vi "Generate mounth year strings.vi"(7 "Dashes?":bool, 11 "seconds since 1904 (default 0 = now)":u32) -> (0 "mmdd":string, 2 "hhmmss_mmdd":string, 3 "Month_year":string)   [LabVIEW 2015]
panel:
  out "Old result":string
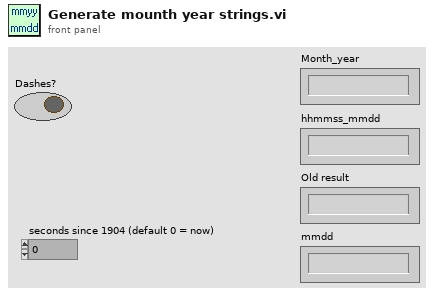
[diagram p1: front panel]
types:
  T1 = typedef "LVDateTimeRec.ctl" = cluster{"fractional second":dbl, "second":i32, "minute":i32, "hour":i32, "day of month":i32, "month":i32, "year":i32, "day of week":i32, "day of year":i32, "DST":i32}
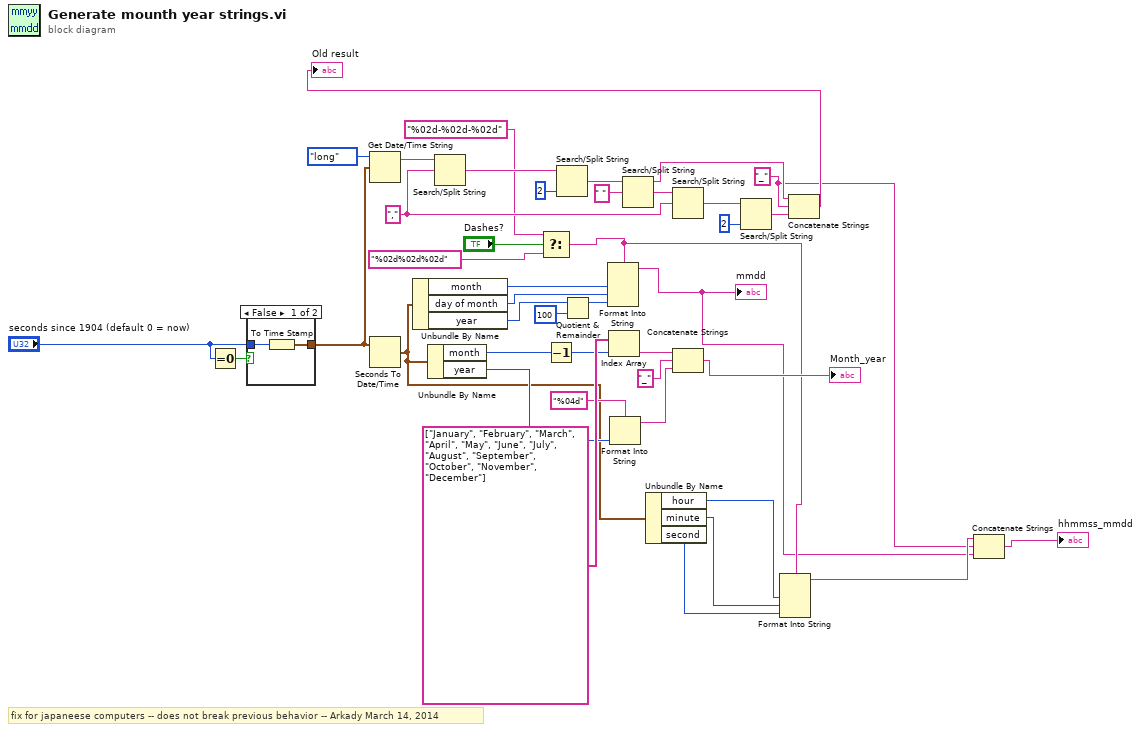
[diagram p0: block diagram]
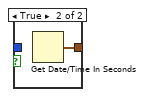
[diagram p2: hidden frame]
diagram:
  w2 = "_" ("substring before char")
  w34 = ","
  # "fix for japaneese computers -- does not break previous behavior -- Arkady March 14, 2014"
  n1 = Equal To 0?(x="seconds since 1904 (default 0 = now)") -> (x = 0?=w31:bool)
  n2 = case shown="False" w31 {
    tunnel: [w43 w45] -> w25
    tunnel: "seconds since 1904 (default 0 = now)" -> [w44 _]
    frame False {
      n3 = To Time Stamp(1:w44) -> (0:w43:timestamp)
    }
    frame True {
      n4 = Get Date/Time In Seconds() -> (seconds since 1Jan1904=w45:timestamp)
    }
  }
  n5 = Get Date/Time String(date format (0)=enum16{"short", "long", "abbreviated"}."long", seconds (now)=w25) -> (date string=w42:string)  [unwired: 2 out]
  n6 = Seconds To Date/Time(time stamp (now)=w25) -> (date time rec=w9:T1)  [unwired: 1 out]
  n7 = Unbundle By Name(w9) -> ("month"=w29:i32, "day of month"=w28:i32, "year"=w13:i32)
  n8 = Unbundle By Name(w9) -> ("month"=w15:i32, "year"=w12:i32)
  n9 = Search/Split String(string=w42, search string/char (-)=w34) -> (match + rest of string=w40:string)  [unwired: 3 out]
  n10 = Select(t="%02d-%02d-%02d", s="Dashes?", f="%02d%02d%02d") -> (s? t:f=w8:string)
  n11 = Decrement(x=w15) -> (x-1=w14:i32)
  n12 = Search/Split String(string=w40, offset (0)=2) -> (match + rest of string=w39:string)  [unwired: 3 out]
  n13 = Quotient & Remainder(x=w13, y=100) -> (x-y*floor(x/y)=w26:i32)  [unwired: 1 out]
  n14 = Format Into String(format string=w8, w29, w28, w26) -> (resulting string=w3:string)  [unwired: 2 in, 1 out]
  "mmdd" <- w3
  n15 = Index Array(array=string[] ["January", "February", "March", "April", "May", "June", "July", "August", "September", "October", "November", "December"], index=w14) -> (element=w18:string)
  n16 = Format Into String(format string="%04d", w12) -> (resulting string=w16:string)  [unwired: 2 in, 1 out]
  n17 = Search/Split String(string=w39, search string/char (-)=" ") -> (substring before match=w32:string, match + rest of string=w36:string)  [unwired: 2 out]
  n18 = Unbundle By Name(w9) -> ("hour"=w7:i32, "minute"=w6:i32, "second"=w5:i32)
  n19 = Search/Split String(string=w36, search string/char (-)=w34) -> (match + rest of string=w33:string)  [unwired: 3 out]
  n20 = Concatenate Strings(w18, "_" ("substring before char"), w16) -> (→"Month_year":string)
  n21 = Search/Split String(string=w33, offset (0)=2) -> (match + rest of string=w37:string)  [unwired: 3 out]
  n22 = Format Into String(format string=w8, w7, w6, w5) -> (resulting string=w4:string)  [unwired: 2 in, 1 out]
  n23 = Concatenate Strings(w32, w2, w37) -> (→"Old result":string)
  n24 = Concatenate Strings(w4, w2, w3) -> (→"hhmmss_mmdd":string)
